vi "Row_Create.vi"(8 "error in (no error)":errorcluster, 10 "StartPoint":T1, 11 "reference in":refnum<class "Row.lvclass">) -> (0 "error out":errorcluster, 3 "reference out":refnum<class "Row.lvclass">)   [LabVIEW 2012, in "Row.lvclass"]
uses:
  Row.lvclass
  Glyph_class/Position.ctl
  Glyph_class/Glyph.lvclass
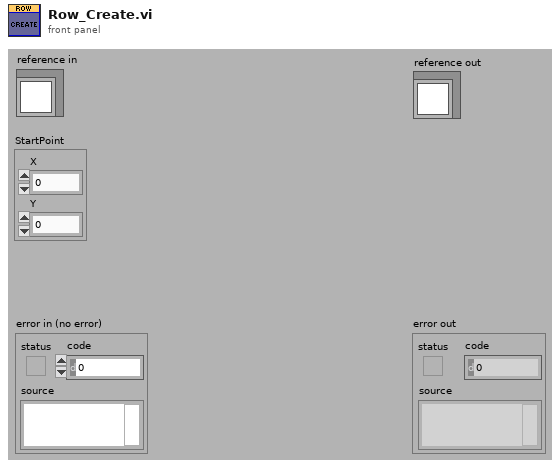
[diagram p1: front panel]
types:
  T1 = typedef "Glyph.lvclass/Position.ctl" = cluster{"X":i32, "Y":i32}
  T2 = typedef "Row.lvclass/ObjectAttributes.ctl" = cluster{"Characters":refnum<class "Character.lvclass">[], "StartPoint":T1, "CharacterSpacing":i32}
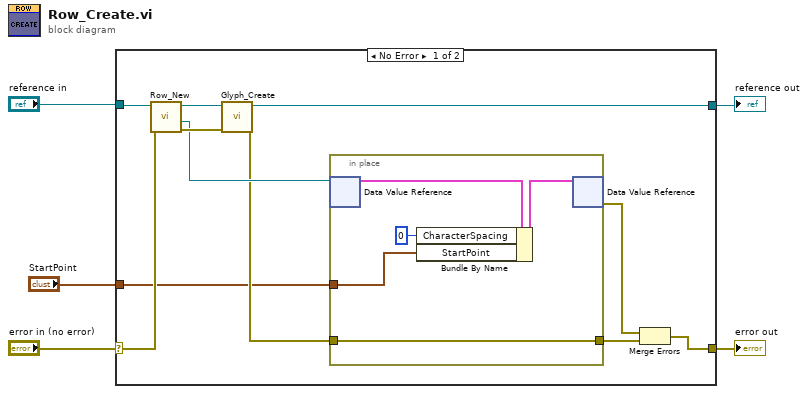
[diagram p0: block diagram]
diagram:
  n1 = case shown="No Error" "error in (no error)" {
    selector: "error in (no error)" -> [w13 w23]
    tunnel: [w11 w23] -> w4
    tunnel: "reference in" -> [w15 w22]
    tunnel: [w10 w22] -> w2
    tunnel: "StartPoint" -> [w6 _]
    frame No Error {
      n2 = call "Row_New.vi"("error in (no error)"=w13, "reference in"=w15) -> ("error out"=w14:errorcluster, "DVRRefOut"=w9:refnum<data-value>, "reference out"=w16:refnum<class "Row.lvclass">)  [unwired: 6 in, 1 out]
      n3 = call "Glyph_Create.vi"("error in (no error)"=w14, "reference in"=w16) -> ("error out"=w8:errorcluster, "reference out"=w10:refnum<class "Row.lvclass">)  [unwired: 8 in]
      n4 = in-place {
        in-place-border: w8 -> [w19]
        in-place-border: [w19] -> w7
        in-place-border: w6 -> [w17]
        n5 = in-place-dvr #1(w9) -> (w20:T2)  [unwired: 1 out]
        n6 = Bundle By Name(cluster=w20, "CharacterSpacing"=0, "StartPoint"=w17) -> (w21:T2)
        n7 = in-place-dvr #1(w21) -> (w12:errorcluster)  [unwired: 1 out]
      }
      n8 = Merge Errors(w12, w7) -> (w11:errorcluster)
    }
    frame Error {
    }
  }
  "error out" <- w4
  "reference out" <- w2
